vi "get stage settings.vi"(8 "error in (no error)":errorcluster, 10 "stage_settings":T1, 11 "id":i32) -> (0 "error out":errorcluster, 2 "stage_settings out":T1, 3 "function return":i32)   [LabVIEW 2012, in "libximc.lvlib"]
doc: "result_t XIMC_API get_stage_settings (device_t id, stage_settings_t* stage_settings);"
uses:
  libximc.lvlib
  libximc.dll
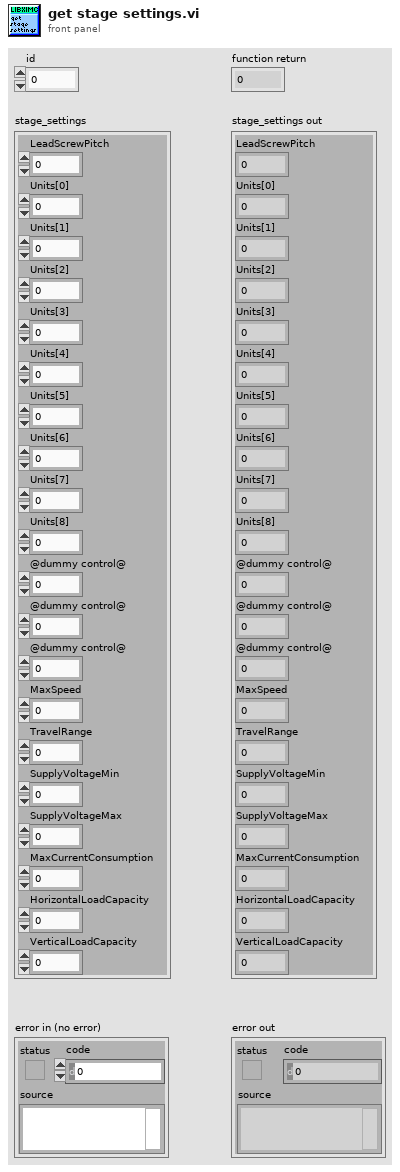
[diagram p1: front panel]
types:
  T1 = cluster{"LeadScrewPitch":sgl, "Units[0]":i8, "Units[1]":i8, "Units[2]":i8, "Units[3]":i8, "Units[4]":i8, "Units[5]":i8, "Units[6]":i8, "Units[7]":i8, "Units[8]":i8, "@dummy control@":i8, "@dummy control@":i8, "@dummy control@":i8, "MaxSpeed":sgl, "TravelRange":sgl, "SupplyVoltageMin":sgl, "SupplyVoltageMax":sgl, "MaxCurrentConsumption":sgl, "HorizontalLoadCapacity":sgl, "VerticalLoadCapacity":sgl}
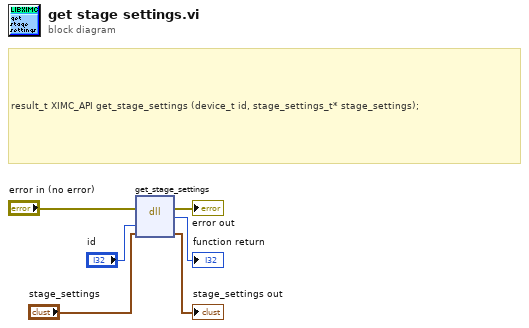
[diagram p0: block diagram]
diagram:
  # "result_t XIMC_API get_stage_settings (device_t id, stage_settings_t* stage_settings);"
  n1 = dll-call lib="C:/Users/Vasily/Att_examples/LabVIEW_example/libximc.*" fn="get_stage_settings"(error in="error in (no error)", "id"="id", "stage_settings"="stage_settings") -> (error out=→"error out":errorcluster, →"function return":i32, "stage_settings"=→"stage_settings out":T1)  [unwired: 3 in, 1 out]
